vi "Choreo_DifferentialSample_IntegrateFunction.vi"(9 "U":T1, 10 "X":T1, 11 "PassedData":variant) -> (0 "Error":bool, 3 "Output":T1)   [LabVIEW 2019, in "ChoreoLib.lvlib"]
uses:
  ChoreoLib.lvlib
  <vilib>/Analysis/Matrix/Datatypes/RealMatrix.ctl
  <vilib>/Rock Robotics/WPI/ThirdParty/JAS_Junk/TrajLib/MatBuilder_Create.vi
  <vilib>/Rock Robotics/WPI/ThirdParty/JAS_Junk/TrajLib/Trajectory_Library.lvlib
  <vilib>/Analysis/Matrix/NI_Matrix.lvlib
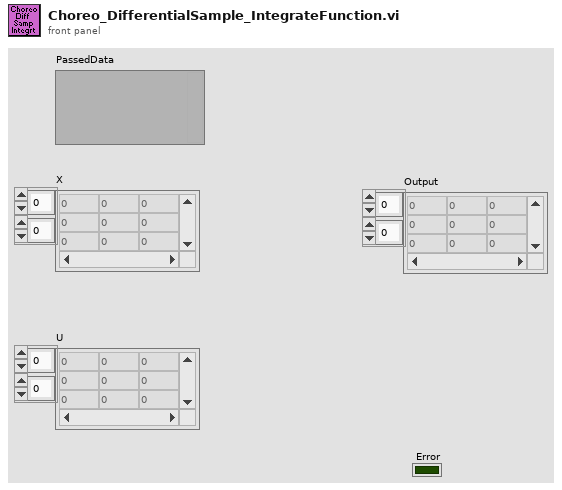
[diagram p1: front panel]
types:
  T1 = typedef "NI_Matrix.lvlib/RealMatrix.ctl" = dbl[][]
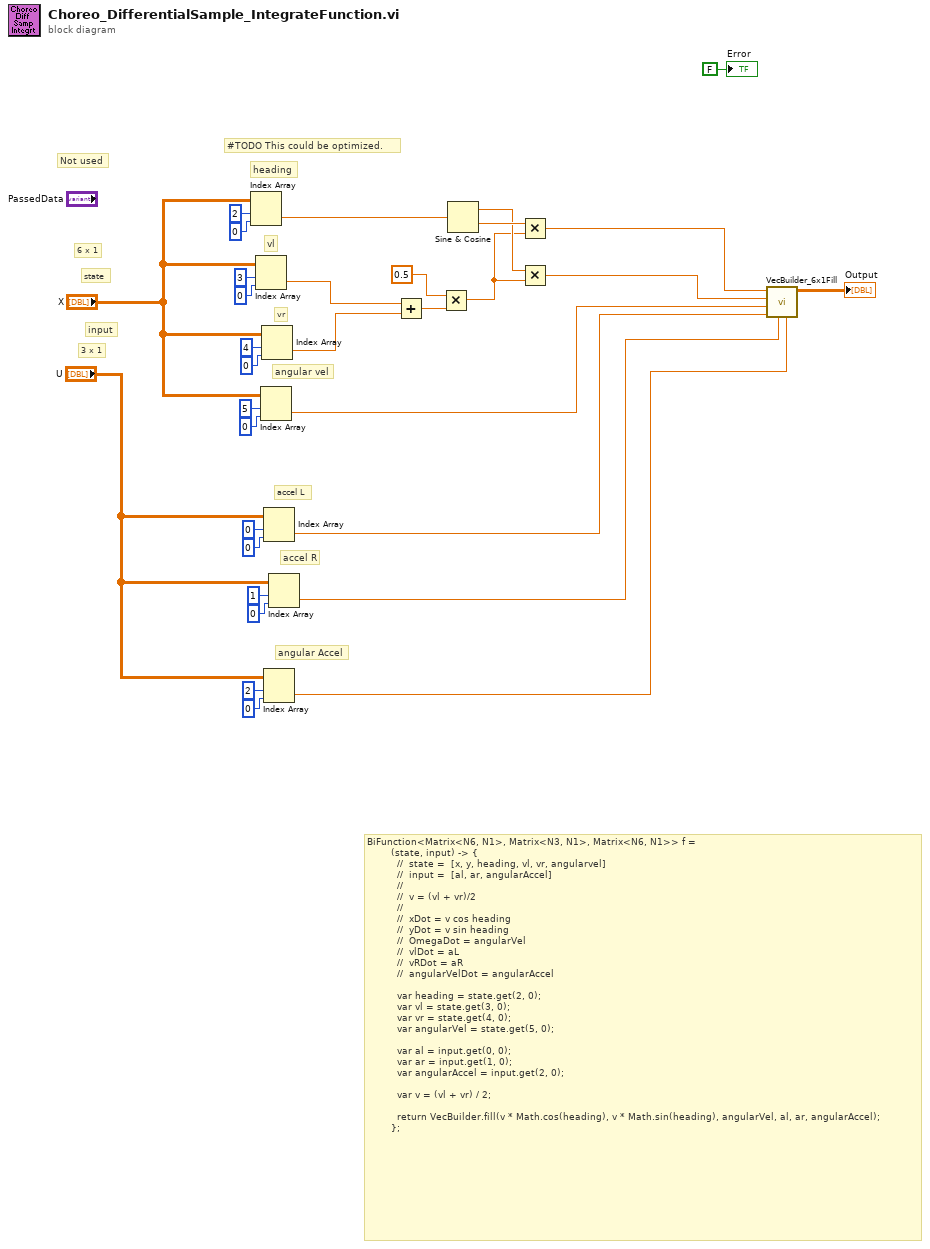
[diagram p0: block diagram]
diagram:
  # "#TODO This could be optimized."
  # "angular Accel"
  # "accel R"
  # "accel L"
  # "input"
  # "state"
  # "angular vel"
  # "vr"
  # "vl"
  # "heading"
  # "Not used"
  # "3 x 1"
  # "6 x 1"
  # "BiFunction<Matrix<N6, N1>, Matrix<N3, N1>, Matrix<N6, N1>> f =\n        (state, input) -> {\n          //  state =  [x, y, heading, vl, vr, angularvel]\n          //  input =  [al, ar, angularAccel]\n          //\n          //  v = (vl + vr)/2\n          //\n          //  xDot = v cos heading\n          //  yDot = v sin heading\n          //  OmegaDot = angularVel\n          //  vlDot = aL\n          //  vRDot = aR\n          //  angularVelDot = angularAccel\n\n          var heading = state.get(2, 0);\n          var vl = state.get(3, 0);\n          var vr = state.get(4, 0);\n          var angularVel = state.get(5, 0);\n\n          var al = input.get(0, 0);\n          var ar = input.get(1, 0);\n          var angularAccel = input.get(2, 0);\n\n          var v = (vl + vr) / 2;\n\n          return VecBuilder.fill(v * Math.cos(heading), v * Math.sin(heading), angularVel, al, ar, angularAccel);\n        };"
  n1 = Index Array(array="X", index (row)=2, index (col)=0) -> (element=w12:dbl)
  n2 = Index Array(array="X", index (row)=3, index (col)=0) -> (element=w14:dbl)
  n3 = Index Array(array="X", index (row)=5, index (col)=0) -> (element=w6:dbl)
  n4 = Index Array(array="X", index (row)=4, index (col)=0) -> (element=w13:dbl)
  n5 = Index Array(array="U", index (row)=0, index (col)=0) -> (element=w5:dbl)
  n6 = Index Array(array="U", index (row)=2, index (col)=0) -> (element=w3:dbl)
  n7 = Index Array(array="U", index (row)=1, index (col)=0) -> (element=w4:dbl)
  n8 = Add(x=w14, y=w13) -> (x+y=w16:dbl)
  n9 = Multiply(x=0.5, y=w16) -> (x*y=w7:dbl)
  n10 = Sine & Cosine(0:w12) -> (1:w8:dbl, 2:w11:dbl)
  n11 = Multiply(x=w11, y=w7) -> (x*y=w10:dbl)
  n12 = Multiply(x=w8, y=w7) -> (x*y=w9:dbl)
  n13 = call <vilib>:"VecBuilder_6x1Fill.vi"("R5"=w3, "R4"=w4, "R3"=w5, "R2"=w6, "R1"=w9, "R0"=w10) -> ("output matrix"=→"Output":T1)  [unwired: 5 in]
  "Error" <- FALSE ("Error")
